vi "Create Value.vi"(8 "error in (no error)":errorcluster, 11 "NT Scalar (Numeric) in":refnum<class "NT Scalar (Numeric).lvclass">) -> (0 "error out":errorcluster, 2 "PV Data out":refnum<class "PV Data.lvclass">, 3 "NT Scalar (Numeric) out":refnum<class "NT Scalar (Numeric).lvclass">)   [LabVIEW 2020, in "PV Access.lvlib" / "PV Data.lvlib" / "NT Scalar (Numeric).lvclass"]
uses:
  NT Scalar (Numeric).lvclass
  C:/Users/eyw68381/source/repos/pvaccess-labview/labview/source/PV Data/NT Scalar/NT Scalar.lvclass
  C:/Users/eyw68381/source/repos/pvaccess-labview/labview/source/PV Data/NT Base/NT Base.lvclass
  PV Data/PV Data.lvclass
  82ca8799-6833-489c-ad76-1514e4833bf9.vi
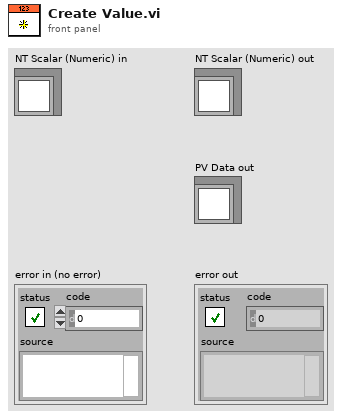
[diagram p1: front panel]
types:
  T1 = typedef "PV Access.lvlib/PV Data.lvlib/Value Fields.ctl" = cluster{"Display":bool, "Control":bool, "Alarm Limits":bool}
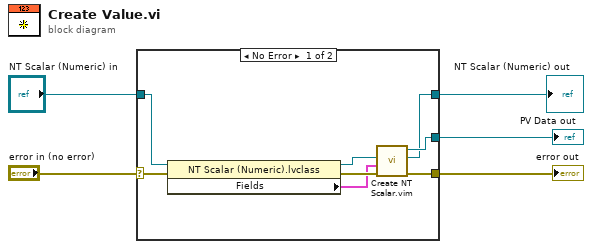
[diagram p0: block diagram]
diagram:
  n1 = case shown="No Error" "error in (no error)" {
    selector: "error in (no error)" -> [w12 w15]
    tunnel: [w10 w15] -> w4
    tunnel: [w6 w14] -> w1
    tunnel: "NT Scalar (Numeric) in" -> [w13 w14]
    tunnel: [w9 _] -> w3
    frame No Error {
      n2 = property class="NT Scalar (Numeric).lvclass"(reference=w13, error in=w12) -> (reference out=w7:refnum<class "NT Scalar (Numeric).lvclass">, error out=w11:errorcluster, "Fields"=w8:T1)
      n3 = call "Create NT Scalar.vim"("error in (no error)"=w11, "fields"=w8, "initial value"=w7) -> ("error out"=w10:errorcluster, "value out"=w6:refnum<class "NT Scalar (Numeric).lvclass">, "PV Data out"=w9:refnum<class "PV Data.lvclass">)  [unwired: 5 in, 1 out]
    }
    frame Error {
    }
  }
  "NT Scalar (Numeric) out" <- w1
  "error out" <- w4
  "PV Data out" <- w3
